vi "abort PS.vi"   [LabVIEW 2020]
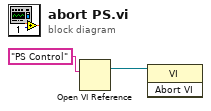
[diagram p0: block diagram]
diagram:
  n1 = Open VI Reference(vi path="PS Control") -> (vi reference=w2:refnum<vi>)  [unwired: 5 in, 1 out]
  n2 = invoke class="VI" method="Abort VI"(reference=w2) -> ()  [unwired: 2 in, 3 out]
